vi "SetSolenoidState.vi"(8 "error in (no error)":errorcluster, 10 "Solenoid On?":bool, 11 "Solenoids in":refnum<class "Solenoids.lvclass">) -> (0 "error out":errorcluster, 3 "Solenoids out":refnum<class "Solenoids.lvclass">)   [LabVIEW 2019, in "Pneumatics control.lvlib" / "Solenoids.lvclass"]
doc: "This VI switches the pneumatic piston from HIGH to LOW depending on the boolean that arrives. If the boolean does not change, and the switching time has elapsed, then it will keep the solenid off."
uses:
  Solenoids.lvclass
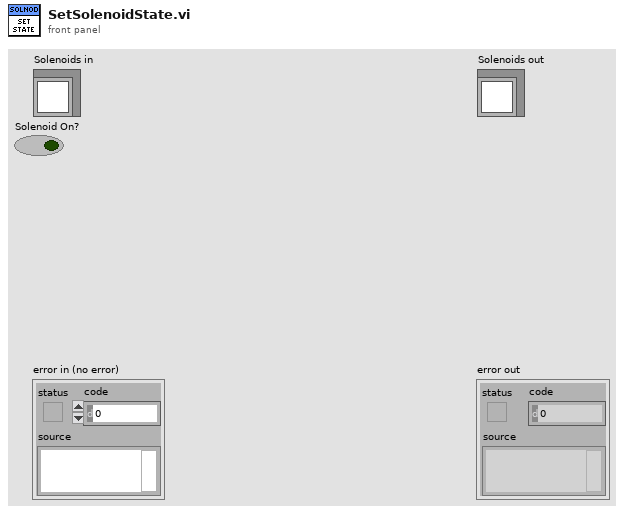
[diagram p1: front panel]
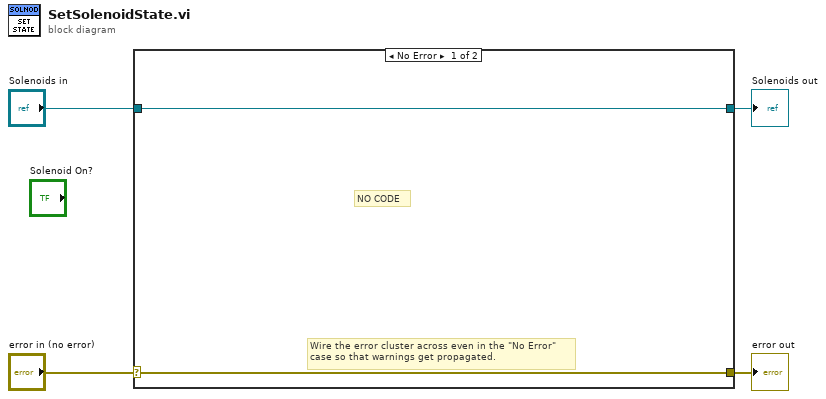
[diagram p0: block diagram]
diagram:
  n1 = case shown="No Error" "error in (no error)" {
    selector: "error in (no error)" -> [w5 w8]
    tunnel: [w5 w8] -> w3
    tunnel: [w6 w7] -> w1
    tunnel: "Solenoids in" -> [w6 w7]
    frame No Error {
      # "NO CODE"
      # "Wire the error cluster across even in the \"No Error\"\ncase so that warnings get propagated."
    }
    frame Error {
    }
  }
  "error out" <- w3
  "Solenoids out" <- w1
